vi "2.1.vi"() -> ()   [LabVIEW 2020]
panel:
  in  "?":bool
  out "Serie de fibonacci":i64[](array[numeric])
  in  "limite":i64
  out "resultado":i64
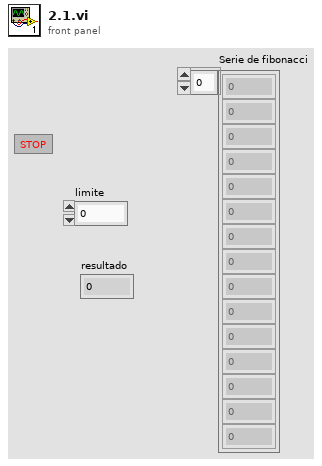
[diagram p1: front panel]
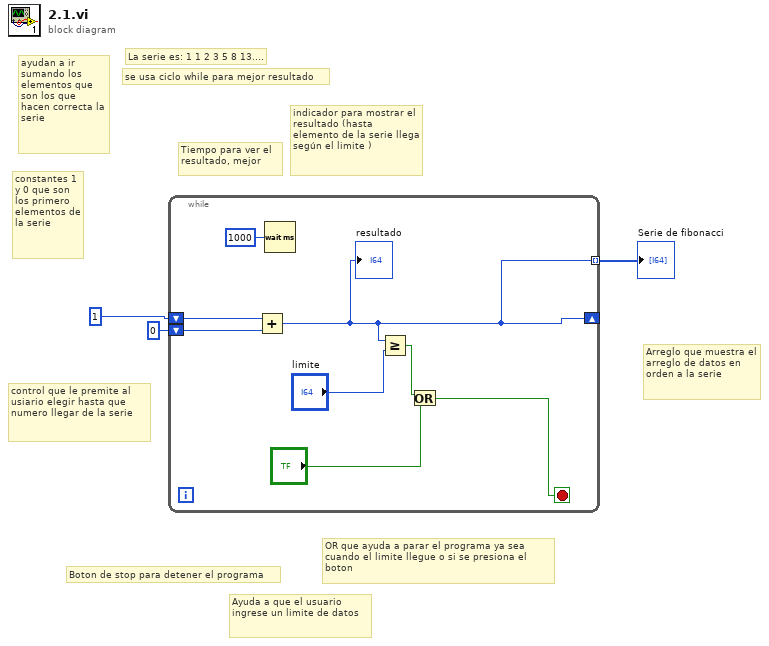
[diagram p0: block diagram]
diagram:
  # "Arreglo que muestra el arreglo de datos en orden a la serie"
  # "Ayuda a que el usuario ingrese un limite de datos"
  # "OR que ayuda a parar el programa ya sea cuando el limite llegue o si se presiona el boton"
  # "ayudan a ir sumando los elementos que son los que hacen correcta la serie"
  # "se usa ciclo while para mejor resultado"
  # "Boton de stop para detener el programa"
  # "control que le premite al usiario elegir hasta que numero llegar de la serie"
  # "constantes 1 y 0 que son los primero elementos de la serie"
  # "Tiempo para ver el \nresultado, mejor"
  # "indicador para mostrar el resultado (hasta \nelemento de la serie llega según el limite )"
  # "La serie es: 1 1 2 3 5 8 13...."
  n1 = while {
    shift-right: [w6] -> _
    shift-left: 1 -> [w11]
    shift-left: 0 -> [w10]
    tunnel: [w6] -> w1 mode=indexing
    stop <- w9 stop-if-true
    n2 = Add(x=w11, y=w10) -> (x+y=w6:i32)
    "resultado" <- w6
    n3 = Wait (ms)(milliseconds to wait=u32 1000) -> ()  [unwired: 1 out]
    n4 = Greater Or Equal?(x=w6, y="limite") -> (x >= y?=w8:bool)
    n5 = Or(x=w8, y="?") -> (x .or. y?=w9:bool)
  }
  "Serie de fibonacci" <- w1
